vi "acq.ImageAccumulator.PL.vi"(6 "loop":i32, 8 "error in":errorcluster, 9 "Dark in":u16[][](array[numeric]), 10 "PL in":u16[][](array[numeric]), 11 "Bright in":u16[][](array[numeric])) -> (0 "error out":errorcluster, 1 "Dark out":u16[][](array[numeric]), 2 "PL out":u16[][](array[numeric]), 3 "Bright out":u16[][](array[numeric]))   [LabVIEW 2020]
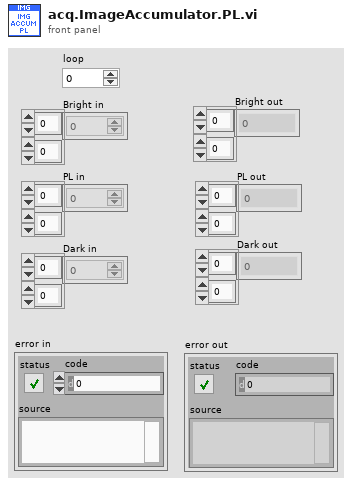
[diagram p1: front panel]
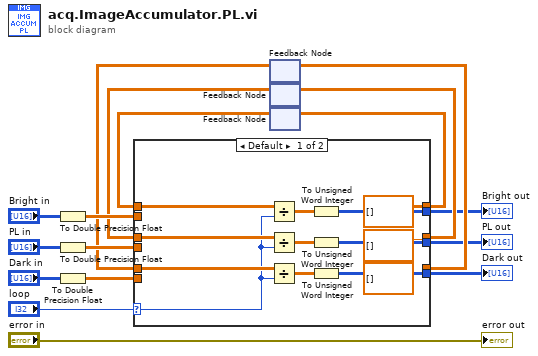
[diagram p0: block diagram]
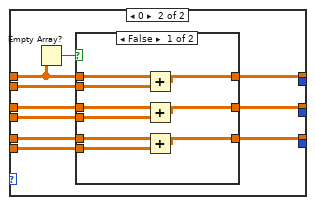
[diagram p2: hidden frame]
diagram:
  n1 = To Double Precision Float(number="Bright in") -> (double precision float=w11:dbl[][])
  n2 = To Double Precision Float(number="PL in") -> (double precision float=w8:dbl[][])
  n3 = To Double Precision Float(number="Dark in") -> (double precision float=w10:dbl[][])
  n4 = feedback #1() -> (w5:dbl[][])  [unwired: 1 in]
  n5 = feedback #2() -> (w6:dbl[][])  [unwired: 1 in]
  n6 = feedback #3() -> (w12:dbl[][])  [unwired: 1 in]
  n7 = case shown="Default" "loop" {
    selector: "loop" -> [w21 _]
    tunnel: w12 -> [w30 w31]
    tunnel: [dbl[][] [] w33] -> w16
    tunnel: w11 -> [_ w40]
    tunnel: w6 -> [w29 w37]
    tunnel: w5 -> [w28 w39]
    tunnel: w10 -> [_ w38]
    tunnel: [dbl[][] [] w35] -> w9
    tunnel: w8 -> [_ w36]
    tunnel: [dbl[][] [] w34] -> w7
    tunnel: [w24 _] -> w4
    tunnel: [w23 _] -> w3
    tunnel: [w22 _] -> w2
    frame Default {
      n8 = Divide(x=w30, y=w21) -> (x/y=w27:dbl[][])
      n9 = Divide(x=w29, y=w21) -> (x/y=w26:dbl[][])
      n10 = Divide(x=w28, y=w21) -> (x/y=w25:dbl[][])
      n11 = To Unsigned Word Integer(number=w27) -> (unsigned 16bit integer=w24:u16[][])
      n12 = To Unsigned Word Integer(number=w26) -> (unsigned 16bit integer=w23:u16[][])
      n13 = To Unsigned Word Integer(number=w25) -> (unsigned 16bit integer=w22:u16[][])
    }
    frame 0 {
      n14 = Empty Array?(array=w31) -> (empty?=w32:bool)
      n15 = case shown="False" w32 {
        tunnel: w40 -> [w49 w52]
        tunnel: w31 -> [w48 _]
        tunnel: w39 -> [w47 _]
        tunnel: w38 -> [w46 w50]
        tunnel: w37 -> [w45 _]
        tunnel: w36 -> [w44 w51]
        tunnel: [w43 w50] -> w35
        tunnel: [w42 w51] -> w34
        tunnel: [w41 w52] -> w33
        frame False {
          n16 = Add(x=w48, y=w49) -> (x+y=w41:dbl[][])
          n17 = Add(x=w45, y=w44) -> (x+y=w42:dbl[][])
          n18 = Add(x=w47, y=w46) -> (x+y=w43:dbl[][])
        }
        frame True {
        }
      }
    }
  }
  "Bright out" <- w4
  "PL out" <- w3
  "Dark out" <- w2
  n19 = feedback-in #1(w9) -> ()
  n20 = feedback-in #2(w7) -> ()
  n21 = feedback-in #3(w16) -> ()
  "error out" <- "error in"
